vi "Dynamic Events- Consumer Producer.vi"() -> ()   [LabVIEW 2021]
panel:
  out "Boolean 2":bool
  out "Slide 2":dbl
  out "String 2":string
  in  "String":string
  in  "Boolean":bool
  in  "Slide":dbl(slide) scale=0.0..10.0
  # "Producer Consumer Using Events"
  # "Consumer"
  # "Producer"
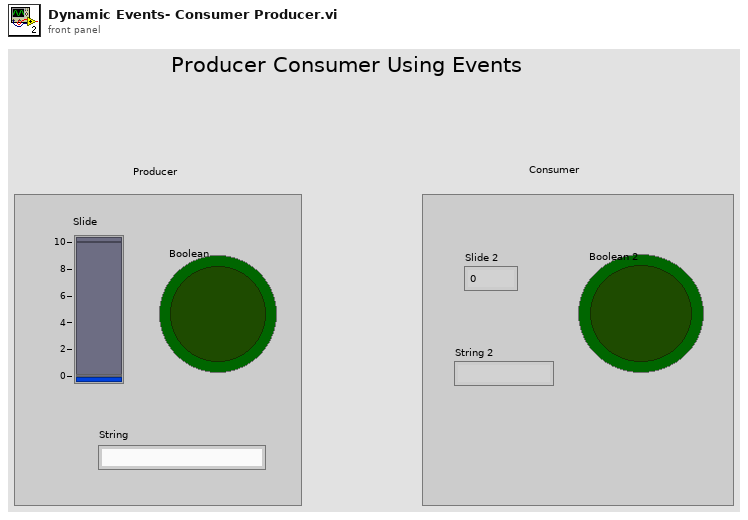
[diagram p1: front panel]
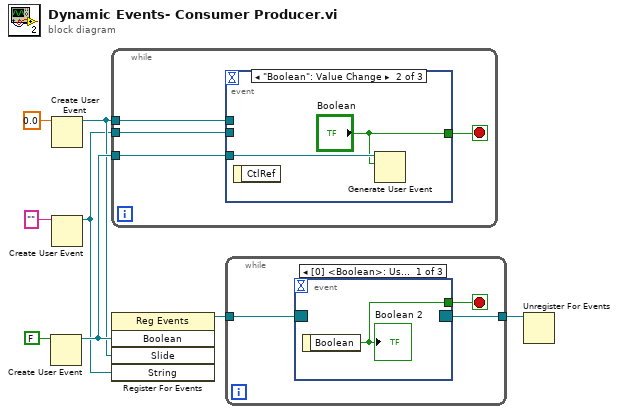
[diagram p0: block diagram]
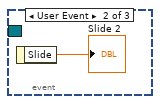
[diagram p2: hidden frame]
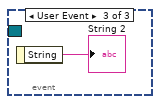
[diagram p3: hidden frame]
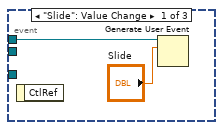
[diagram p4: hidden frame]
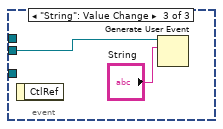
[diagram p5: hidden frame]
diagram:
  n1 = Create User Event(user event datatype=FALSE ("Boolean")) -> (user event=w5:refnum<user-event>)  [unwired: 1 in, 1 out]
  n2 = Create User Event(user event datatype=0.0 ("Slide")) -> (user event=w4:refnum<user-event>)  [unwired: 1 in, 1 out]
  n3 = Create User Event(user event datatype="" ("String")) -> (user event=w3:refnum<user-event>)  [unwired: 1 in, 1 out]
  n4 = while {
    tunnel: w5 -> [w12]
    tunnel: w4 -> [w11]
    tunnel: w3 -> [w10]
    stop <- w9 stop-if-true
    n5 = event shown="[1] \"Boolean\": Value Change" {
      selector: _ -> [_ _ _]
      dyn-events: _ -> [_ _ _]
      timeout: _ -> [_ _ _]
      tunnel: w12 -> [_ w16 _]
      tunnel: w11 -> [w14 _ _]
      tunnel: w10 -> [_ _ w18]
      tunnel: [_ "Boolean" _] -> w9
      event "Slide": Value Change {
        n6 = event-data() -> ()  [unwired: 1 in, 1 out]
        n7 = Generate User Event(user event=w14, event data cluster="Slide") -> ()  [unwired: 2 in, 2 out]
      }
      event "Boolean": Value Change {
        n8 = event-data() -> ()  [unwired: 1 in, 1 out]
        n9 = Generate User Event(user event=w16, event data cluster="Boolean") -> ()  [unwired: 2 in, 2 out]
      }
      event "String": Value Change {
        n10 = event-data() -> ()  [unwired: 1 in, 1 out]
        n11 = Generate User Event(user event=w18, event data cluster="String") -> ()  [unwired: 2 in, 2 out]
      }
    }
  }
  n12 = register-events(w5, w4, w3) -> (reference out=w2:refnum<event-registration>)  [unwired: 2 in, 1 out]
  n13 = while {
    tunnel: w2 -> [w20]
    tunnel: [w21] -> w1
    stop <- w19 stop-if-true
    n14 = event shown="[0] <Boolean>: User Event" {
      selector: w20 -> [_ _ _]
      dyn-events: [_ _ _] -> w21
      timeout: _ -> [_ _ _]
      tunnel: [w22 _ _] -> w19
      event User Event {
        n15 = event-data() -> ("Boolean"=w22:bool)  [unwired: 1 in]
        "Boolean 2" <- w22
      }
      event User Event {
        n16 = event-data() -> ("Slide"=→"Slide 2":dbl)  [unwired: 1 in]
      }
      event User Event {
        n17 = event-data() -> ("String"=→"String 2":string)  [unwired: 1 in]
      }
    }
  }
  n18 = Unregister For Events(event registration refnum=w1) -> ()  [unwired: 1 in, 1 out]
